vi "LPD_ASCII String to Hex Byte Array.vi"(10 "String":string="000102030405060708") -> (2 "Hex Byte Array":u8[](array[numeric]) format="%02x")   [LabVIEW 2009]
doc: "LPD_ASCII String to Hex Byte Array.vi\n\n<B>Description:</B>\nThis VI converts an ASCII string to the equivalent Hex byte array.\n\n<B>Inputs:</B>\nString - The string to convert into a Hex byte array.\n\n<B>Outputs:</B>\n\nHex Byte Array - Output Hex byte array.\n\n\nLogicPD, Inc\nwww.logicpd.com"
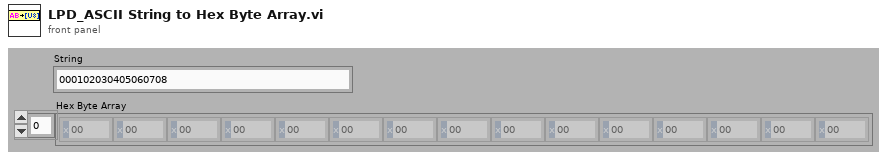
[diagram p1: front panel]
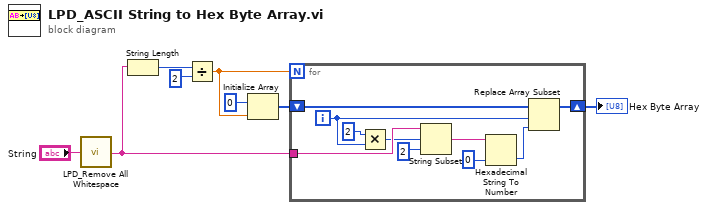
[diagram p0: block diagram]
diagram:
  n1 = call "LPD_Remove All Whitespace.vi"("String"="String") -> ("String out"=w2:string)  [unwired: 8 in]
  n2 = String Length(string=w2) -> (length=w5:i32)
  n3 = Divide(x=w5, y=2) -> (x/y=w7:dbl)
  n4 = Initialize Array(u8 0 ("dimension size"), w7) -> (w8:u8[])
  n5 = for {
    N: w7 -> [_]
    tunnel: w2 -> [w18]
    shift-right: [w9] -> w3
    shift-left: w8 -> [w14]
    i -> [w13]
    n6 = Multiply(x=2, y=w13) -> (x*y=w16:i32)
    n7 = String Subset(string=w18, offset (0)=w16, length (rest)=2 ("length (rest)")) -> (substring=w12:string)
    n8 = Hexadecimal String To Number(string=w12, default (0uL)=u8 0 ("default (0 U32)")) -> (number=w10:u8)  [unwired: 1 in, 1 out]
    n9 = Replace Array Subset(array=w14, new element=w10, index=w13) -> (w9:u8[])
  }
  "Hex Byte Array" <- w3
